vi "Canteen selection.vi"() -> ()   [LabVIEW 2017]
panel:
  in  "Boolean":bool
  in  "Array 4":bool[](array[boolean])=[TRUE, TRUE, TRUE, TRUE]
  in  "Array 3":bool[](array[boolean])=[TRUE, TRUE, TRUE, TRUE, TRUE, TRUE, TRUE, TRUE, TRUE, TRUE, TRUE, TRUE, TRUE]
  in  "Array 2":bool[](array[boolean])=[TRUE, TRUE, TRUE, TRUE]
  in  "Array":bool[](array[boolean])=[FALSE, FALSE, FALSE, FALSE, FALSE, FALSE, FALSE, FALSE, FALSE, FALSE, FALSE, TRUE, TRUE]
  out "String":string
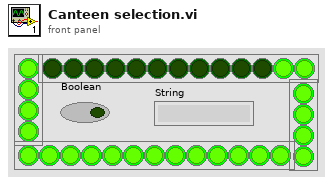
[diagram p1: front panel]
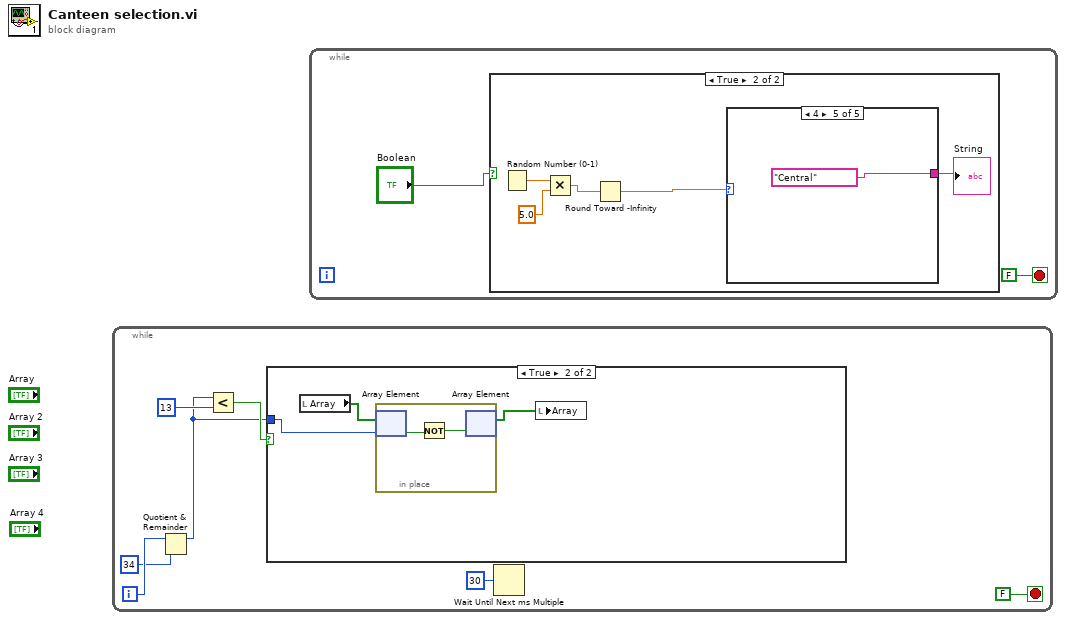
[diagram p0: block diagram]
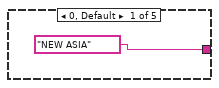
[diagram p3: hidden frame]
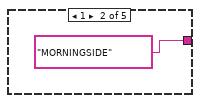
[diagram p4: hidden frame]
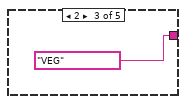
[diagram p5: hidden frame]
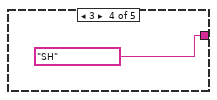
[diagram p6: hidden frame]
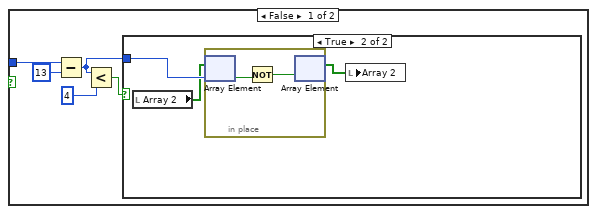
[diagram p7: hidden frame]
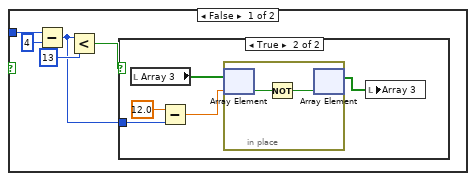
[diagram p8: hidden frame]
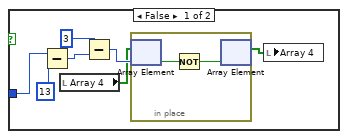
[diagram p9: hidden frame]
diagram:
  n1 = while {
    i -> [w6]
    stop <- FALSE stop-if-true
    n2 = Quotient & Remainder(x=w6, y=34) -> (x-y*floor(x/y)=w2:i32)  [unwired: 1 out]
    n3 = Less?(x=w2, y=13) -> (x < y?=w3:bool)
    n4 = case shown="True" w3 {
      tunnel: w2 -> [w12 w41]
      frame False {
        n5 = Subtract(x=w12, y=13) -> (x-y=w8:i32)
        n6 = Less?(x=w8, y=4) -> (x < y?=w9:bool)
        n7 = case shown="True" w9 {
          tunnel: w8 -> [w17 w36]
          frame False {
            n8 = Subtract(x=w17, y=4) -> (x-y=w13:i32)
            n9 = Less?(x=w13, y=13) -> (x < y?=w14:bool)
            n10 = case shown="True" w14 {
              tunnel: w13 -> [w24 w30]
              frame False {
                n11 = Subtract(x=w24, y=13) -> (x-y=w22:i32)
                n12 = local read "Array 4"() -> (w19:bool[])
                n13 = Subtract(x=3, y=w22) -> (x-y=w20:i32)
                n14 = in-place {
                  n15 = in-place-array #1(w19, w20) -> (w26:bool)
                  n16 = Not(x=w26) -> (.not. x?=w25:bool)
                  n17 = in-place-array #1(w25) -> (w18:bool[])  [unwired: 1 out]
                }
                n18 = local write "Array 4"(w18) -> ()
              }
              frame True {
                n19 = local read "Array 3"() -> (w28:bool[])
                n20 = Subtract(x=12.0, y=w30) -> (x-y=w29:dbl)
                n21 = in-place {
                  n22 = in-place-array #2(w28, w29) -> (w33:bool)
                  n23 = Not(x=w33) -> (.not. x?=w32:bool)
                  n24 = in-place-array #2(w32) -> (w27:bool[])  [unwired: 1 out]
                }
                n25 = local write "Array 3"(w27) -> ()
              }
            }
          }
          frame True {
            n26 = local read "Array 2"() -> (w35:bool[])
            n27 = in-place {
              n28 = in-place-array #3(w35, w36) -> (w38:bool)
              n29 = Not(x=w38) -> (.not. x?=w37:bool)
              n30 = in-place-array #3(w37) -> (w34:bool[])  [unwired: 1 out]
            }
            n31 = local write "Array 2"(w34) -> ()
          }
        }
      }
      frame True {
        n32 = local read "Array"() -> (w40:bool[])
        n33 = in-place {
          n34 = in-place-array #4(w40, w41) -> (w43:bool)
          n35 = Not(x=w43) -> (.not. x?=w42:bool)
          n36 = in-place-array #4(w42) -> (w39:bool[])  [unwired: 1 out]
        }
        n37 = local write "Array"(w39) -> ()
      }
    }
    n38 = Wait Until Next ms Multiple(millisecond multiple=u32 30) -> ()  [unwired: 1 out]
  }
  n39 = while {
    stop <- FALSE stop-if-true
    n40 = case shown="True" "Boolean" {
      frame False {
      }
      frame True {
        n41 = Random Number (0-1)() -> (number: 0 to 1=w50:dbl)
        n42 = Multiply(x=w50, y=5.0) -> (x*y=w48:dbl)
        n43 = Round Toward -Infinity(1:w48) -> (0:w47:dbl)
        n44 = case shown="4" w47 {
          tunnel: ["NEW ASIA" "MORNINGSIDE" "VEG" "SH" "Central"] -> w46
          frame 0, Default {
          }
          frame 1 {
          }
          frame 2 {
          }
          frame 3 {
          }
          frame 4 {
          }
        }
        "String" <- w46
      }
    }
  }
